vi "set ramp rate.vi"(8 "error in (no error)":errorcluster, 9 "Ramp rate (3500 Gs/min)":dbl[unit]=0.005833333333333334, 11 "VISA session":refnum<visa-resource-name>) -> (0 "error out":errorcluster, 3 "dup VISA session":refnum<visa-resource-name>)   [LabVIEW 2017]
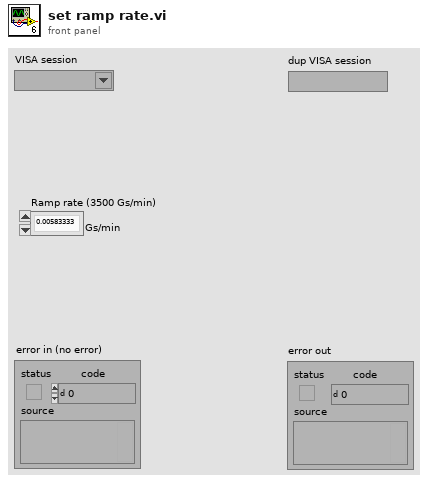
[diagram p1: front panel]
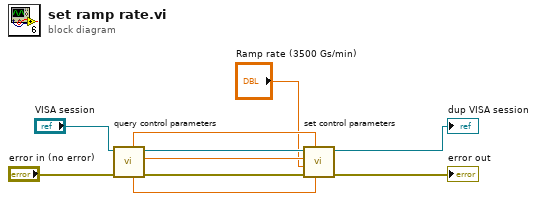
[diagram p0: block diagram]
diagram:
  n1 = call "query control parameters.vi"("error in (no error)"="error in (no error)", "VISA session"="VISA session") -> ("error out"=w6:errorcluster, "Integral"=w10:dbl[unit], "dup VISA session"=w7:refnum<visa-resource-name>, "Control slope limit"=w8:dbl[unit], "Proportional"=w9:dbl)  [unwired: 4 in, 1 out]
  n2 = call "set control parameters.vi"("Control slope limit (10 V/min)"=w8, "Proportional (10)"=w9, "error in (no error)"=w6, "Ramp rate (3500 Gs/min)"="Ramp rate (3500 Gs/min)", "Integral (1 s)"=w10, "VISA session"=w7) -> ("error out"=→"error out":errorcluster, "dup VISA session"=→"dup VISA session":refnum<visa-resource-name>)  [unwired: 4 in]
